vi "MaxContourCount.vi"(3 "Maximum\nContour\nCount":u32 caption="Maximum Contour Count") -> (0 "OK":bool, 1 "New Maximum Contour Count":u32)   [LabVIEW 2009]
panel:
  in  "Cancel Button":bool
  in  "OK Button":bool
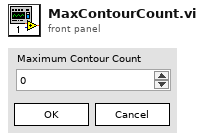
[diagram p1: front panel]
types:
  T1 = enum32{"Invalid", "Standard", "Closed", "Hidden", "Minimized", "Maximized"}
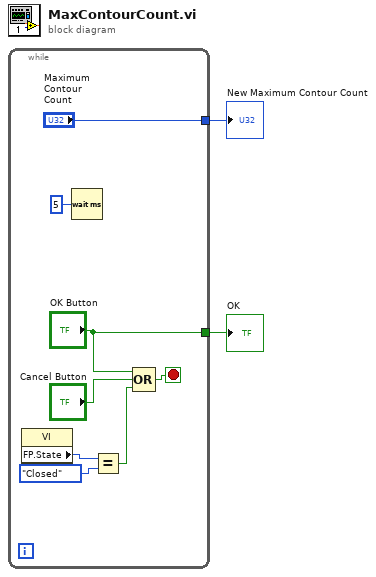
[diagram p0: block diagram]
diagram:
  n1 = while {
    tunnel: ["Maximum\nContour\nCount"] -> w2
    tunnel: ["OK Button"] -> w1
    stop <- w10 stop-if-true
    n2 = property class="VI"() -> ("FP.State"=w6:T1)  [unwired: 2 in, 2 out]
    n3 = Wait (ms)(milliseconds to wait=u32 5) -> ()  [unwired: 1 out]
    n4 = Equal?(x=w6, y=T1."Closed") -> (x = y?=w4:bool)
    n5 = Compound Arithmetic op=OR("OK Button", "Cancel Button", w4) -> (w10:bool)
  }
  "New Maximum Contour Count" <- w2
  "OK" <- w1
